vi "GetProtectedEvent.vi"(8 "error in (no error)":errorcluster, 11 "JKI SMO in":refnum<class "JKI SMO.lvclass">) -> (0 "error out":errorcluster, 2 "Protected Events":T1, 3 "JKI SMO out":refnum<class "JKI SMO.lvclass">)   [LabVIEW 2013, in "JKI SMO.lvclass"]
doc: "Retuns a cluster of Protected User Events for the JKI SMO.\n\n---------------------------------------------------------------\nJKI State Machine Objects™\nhttp://jki.net/state-machine-objects/\nCopyright (C) 2005-2015, JKI <info@jki.net>\nALL RIGHTS RESERVED"
uses:
  JKI SMO.lvclass
  Typedefs/ProtectedEvents--Cluster.ctl
  Typedefs/StopProcessEventData--Cluster.ctl
  Typedefs/AbortProcessEventData--Cluster.ctl
  JKI SMO.lvclass/JKI SMO.ctl
panel:
  # "For instructions on how to use the JKI State Machine Objects, examples and video tutorials, visit:\nhttp://jki.net/state-machine-objects/\n\nJKI State Machine Objects™\nhttp://jki.net/state-machine-objects/\nCopyright (C) 2005-2015, JKI <info@jki.net>\nALL RIGHTS RESERVED"
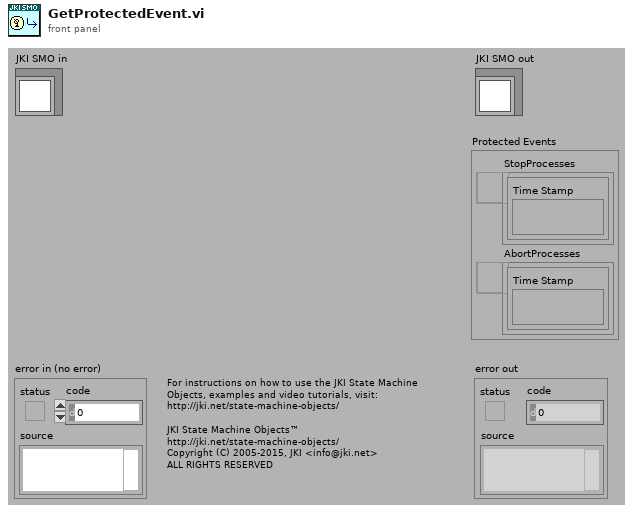
[diagram p1: front panel]
types:
  T1 = typedef "JKI SMO.lvclass/ProtectedEvents--Cluster.ctl" = cluster{"StopProcesses":refnum<user-event>, "AbortProcesses":refnum<user-event>}
  T2 = typedef "pSubSystem.lvclass/pSubSystem.PrivateData--Cluster.ctl" = cluster{"Processes Clone VI Ref [ ]":refnum<vi>[], "Processes Clone Name [ ]":string[], "Process Sync RendezVous":T3, "Protected Events":T4}
  T3 = typedef "Rendezvous RefNum" = refnum<k1>
  T4 = typedef "pSubSystem.lvclass/pSubSystem.ProtectedEvents--Cluster.ctl" = cluster{"StopProcesses":refnum<user-event>, "AbortProcesses":refnum<user-event>}
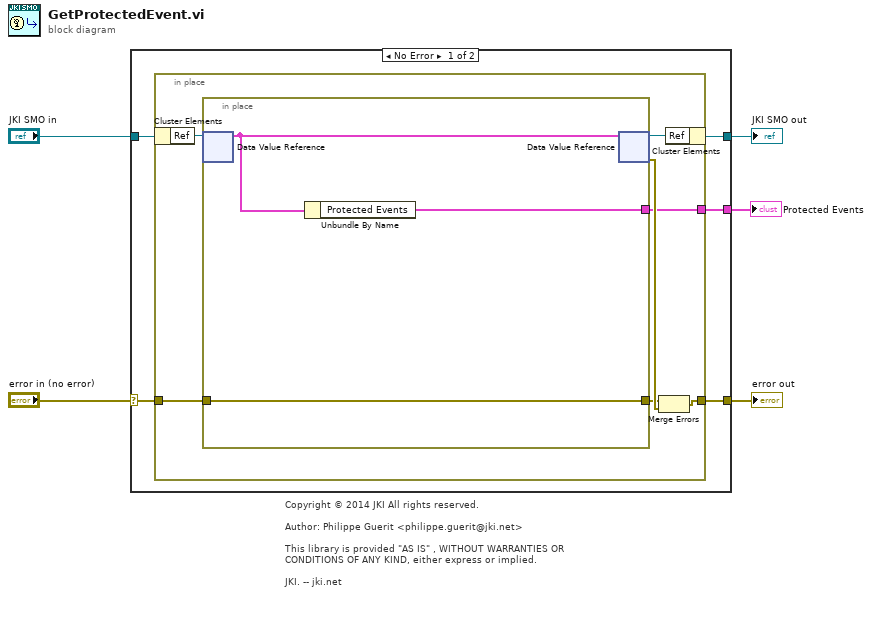
[diagram p0: block diagram]
diagram:
  # "Copyright © 2014 JKI All rights reserved.\n\nAuthor: Philippe Guerit <philippe.guerit@jki.net>\n\nThis library is provided \"AS IS\" , WITHOUT WARRANTIES OR \nCONDITIONS OF ANY KIND, either express or implied.\n\nJKI. -- jki.net"
  n1 = case shown="No Error" "error in (no error)" {
    selector: "error in (no error)" -> [w9 w22]
    tunnel: [w8 w22] -> w4
    tunnel: [w7 w21] -> w2
    tunnel: "JKI SMO in" -> [w10 w21]
    tunnel: [w6 _] -> w1
    frame No Error {
      n2 = in-place {
        in-place-border: w9 -> [w16]
        in-place-border: [w13] -> w8
        in-place-border: [w11] -> w6
        n3 = in-place-cluster #1(w10) -> ("Ref"=w17:refnum<data-value>)
        n4 = in-place {
          in-place-border: w16 -> [w19]
          in-place-border: [w19] -> w14
          in-place-border: [w18] -> w11
          n5 = in-place-dvr #2(w17) -> (w20:T2)  [unwired: 1 out]
          n6 = Unbundle By Name(w20) -> ("Protected Events"=w18:T4)
          n7 = in-place-dvr #2(w20) -> (w12:refnum<data-value>, w15:errorcluster)
        }
        n8 = Merge Errors(w14, w15) -> (w13:errorcluster)
        n9 = in-place-cluster #1("Ref"=w12) -> (w7:refnum<class "JKI SMO.lvclass">)
      }
    }
    frame Error {
    }
  }
  "error out" <- w4
  "JKI SMO out" <- w2
  "Protected Events" <- w1
